vi "Resonator_response.vi"() -> ()   [LabVIEW 2020]
uses:
  <vilib>/Utility/file.llb/Write Delimited Spreadsheet (DBL).vi
  <instrlib>/Keysight PNA Series/Keysight PNA Series.lvlib
panel:
  out "State":T1(ring)=enum."Close"
  in  "PNA_control":T2={"Channel (1)"=1, "Start Frequency (Hz)"=6168700000.0, "Stop Frequency (Hz)"=6170700000.0, "Sweep Points (201)"=201, "Sweep Type (0: Linear)"=0, "Sweep Generation (1: Analog)"=1, "Bandwidth (Hz)"=100.0, "Average Count (1)"=200, "Enable Average "=TRUE, "Power"={"Attenuation (0 dB)"=0.0, "Power Level (0 dBm)"=-50.0, "Enable Auto Attenuation"=TRUE, "Enable RF Power"=TRUE, "Enable Power Slope"=FALSE, "Port (1)"=1, "Power Slope (0 dB/GHz)"=0.0}, "Enable Reduce IF Bandwidth "=TRUE, "Electrical delay"={"Unit (0: Meter)"=0, "Waveguide Cutoff Frequency (Hz)"=45000000.0, "Distance (0)"=0.0, "Medium "=0, "Delay (0 s)"=0.0}, "Measurement name"=["CH1_S12", "CH1_S22"], "Measurement Parameters (S11)"=["S12", "S22"]} {"Electrical delay"."Medium" items=["Coaxial", "Waveguide"]; "Electrical delay"."Unit (0: Meter)" items=["Meter", "Feet", "Inch"]; "Sweep Generation (1: Analog)" items=["Stepped", "Analog"]; "Sweep Type (0: Linear)" items=["Linear", "Logarithmic", "Power", "CW", "Segment", "Phase"]; "Stop Frequency (Hz)" format="%#_8g"; "Start Frequency (Hz)" format="%#_8g"}
  in  "Visa_Cluster":T3={"VNA visa"="GPIB0::16::INSTR", "MG369x visa"="GPIB0::8::INSTR", "Yokogawa visa"="GPIB0::1::INSTR"}
  in  "Save file path":path=path "D:/Sheng-Xiang_Lin/JPA_cooldown14/Fourth_resonator_dispersive_shift"
  in  "File_name":string="qubit"
  in  "Save?":bool=TRUE
  in  "Display format 1-2":T4={"Display Format 2"=3, "Display Format 1"=1} {"Display Format 1" items=["Magnitude Linear", "Magnitude Logarithmic", "Phase", "Unwrapped phase", "Imaginary", "Real", "Polar", "Smith Chart", "Smith Admittance", "SWR", "Group Delay", "Kelvin", "Fahrenheit", "Celsius"]; "Display Format 2" items=["Magnitude Linear", "Magnitude Logarithmic", "Phase", "Unwrapped phase", "Imaginary", "Real", "Polar", "Smith Chart", "Smith Admittance", "SWR", "Group Delay", "Kelvin", "Fahrenheit", "Celsius"]}
  in  "VNA_force_stop":bool
  out "average_times":i32=19
  in  "wait?":bool
  out "Magnitude":dbl[](array[numeric])=[-23.6737670898, -23.7385673523, -23.8055305481, -23.8746070862, -23.9425754547, -24.0142669678, -24.086517334, -24.1621208191, -24.2412757874, -24.3240642548, -24.410150528, -24.4976882935, -24.5875720978, -24.6802349091, -24.7777881622, -24.8763828278, -24.979177475, -25.0872688293, -25.2037525177, -25.3233108521, -25.4416027069, -25.5639820099, -25.704668045, -25.8504219055, -25.9997329712, -26.1532783508, -26.310962677, -26.474363327, -26.6452636719, -26.8241043091, -27.0116844177, -27.2097969055, -27.4203968048, -27.6485824585, -27.8864917755, -28.1318359375, -28.3951377869, -28.6704406738, -28.9638710022, -29.2743930817, -29.603849411, -29.9671974182, -30.3672046661, -30.7709980011, -31.1941585541, -31.6535701752, -32.1623039246, -32.7356109619, -33.3391723633, -34.0166893005, -34.7504501343, -35.5710372925, -36.4783821106, -37.4738388062, -38.6434822083, -40.0588035583, -41.7861747742, -43.9644699097, -46.8876876831, -51.4030303955, -60.4928474426, -57.0826530457, -49.7821121216, -45.7269706726, -42.9327430725, -40.7999610901, -39.0918464661, -37.6644554138, -36.410900116, -35.3036689758, -34.3229827881, -33.4435920715, -32.6499824524, -31.9220294952, -31.2542266846, -30.6332588196, -30.0641708374, -29.5344314575, -29.0330276489, -28.5691413879, -28.1316604614, -27.7197036743, -27.3364849091, -26.9709949493, -26.6234302521, -26.288225174, -25.977640152, -25.6853923798, -25.4085998535, -25.1478462219, -24.8998317719, -24.6655807495, -24.4424247742, -24.2275295258, -24.0214290619, -23.8225841522, -23.63697052, -23.4580116272, -23.3001346588, -23.1510028839, -23.0076026917, -22.8655033112, -22.7290058136, -22.5987110138, -22.4831619263, -22.3689022064, -22.2600975037, -22.1564464569, -22.0540332794, -21.9569740295, -21.8669834137, -21.7826919556, -21.7002334595, -21.6209335327, -21.5461406708, -21.4741287231, -21.4073295593, -21.3435554504, -21.2839221954, -21.2248191833, -21.1635513306, -21.1088104248, -21.0579814911, -21.0078163147, -20.9615936279, -20.9172554016, -20.8747119904, -20.833404541, -20.7956390381, -20.759349823, -20.7250919342, -20.6904773712, -20.6576309204, -20.6262359619, -20.5970096588, -20.5672588348, -20.5403385162, -20.5139713287, -20.4889431, -20.4652805328, -20.440788269, -20.4182872772, -20.3972473145, -20.3769702911, -20.3574924469, -20.338842392, -20.3210716248, -20.3047962189, -20.2892684937, -20.2742462158, -20.2597618103, -20.2454681396, -20.232049942, -20.2189407349, -20.2070941925, -20.1947593689, -20.1833267212, -20.1720867157, -20.1617012024, -20.1521492004, -20.1428623199, -20.1335334778, -20.1245746613, -20.1160011292, -20.1077804565, -20.0995311737, -20.0921134949, -20.0842552185, -20.0772380829, -20.0709438324, -20.0642986298, -20.0582752228, -20.0526847839, -20.0474853516, -20.0421714783, -20.0368518829, -20.0318584442, -20.0270271301, -20.0223388672, -20.0181751251, -20.0138206482, -20.0099639893, -20.0064086914, -20.0029449463, -19.9997406006, -19.9968338013, -19.993806839, -19.9911708832, -19.9880523682, -19.9856872559, -19.9832305908, -19.9805030823, -19.9782714844, -19.9759674072, -19.9742794037, -19.9721908569, -19.970664978, -19.9689235687, -19.9670543671, -19.9657402039, -19.9643135071] format="%#_8g"
  in  "Leave_pend":bool
  in  "Current_Value":T5={"Ch1 Intensity Graph"=array201x26[5226 elements], "Freq_Array"=array[201 elements], "Ch2 Intensity Graph"=array201x26[5226 elements], "Ch1"={"Magnitude"=array[201 elements], "Phase"=array[201 elements]}, "Ch2"={"Magnitude"=array[201 elements], "Phase"=array[201 elements]}, "Signal_power (dBm)"=2.0}
  in  "Limit_Cluster":T6={"Current_or_voltage_limit"=3.0, "Micro_freq_limit (GHz)"=4.71, "Micro_power_limit (dBm)"=0.0}
  in  "Force_stop":bool
  in  "Increment cluster":T7={"Yoko_Increment"=0.01, "Micro_Increment (GHz)"=0.0002, "Micro_power_inc (dBm)"=2.0}
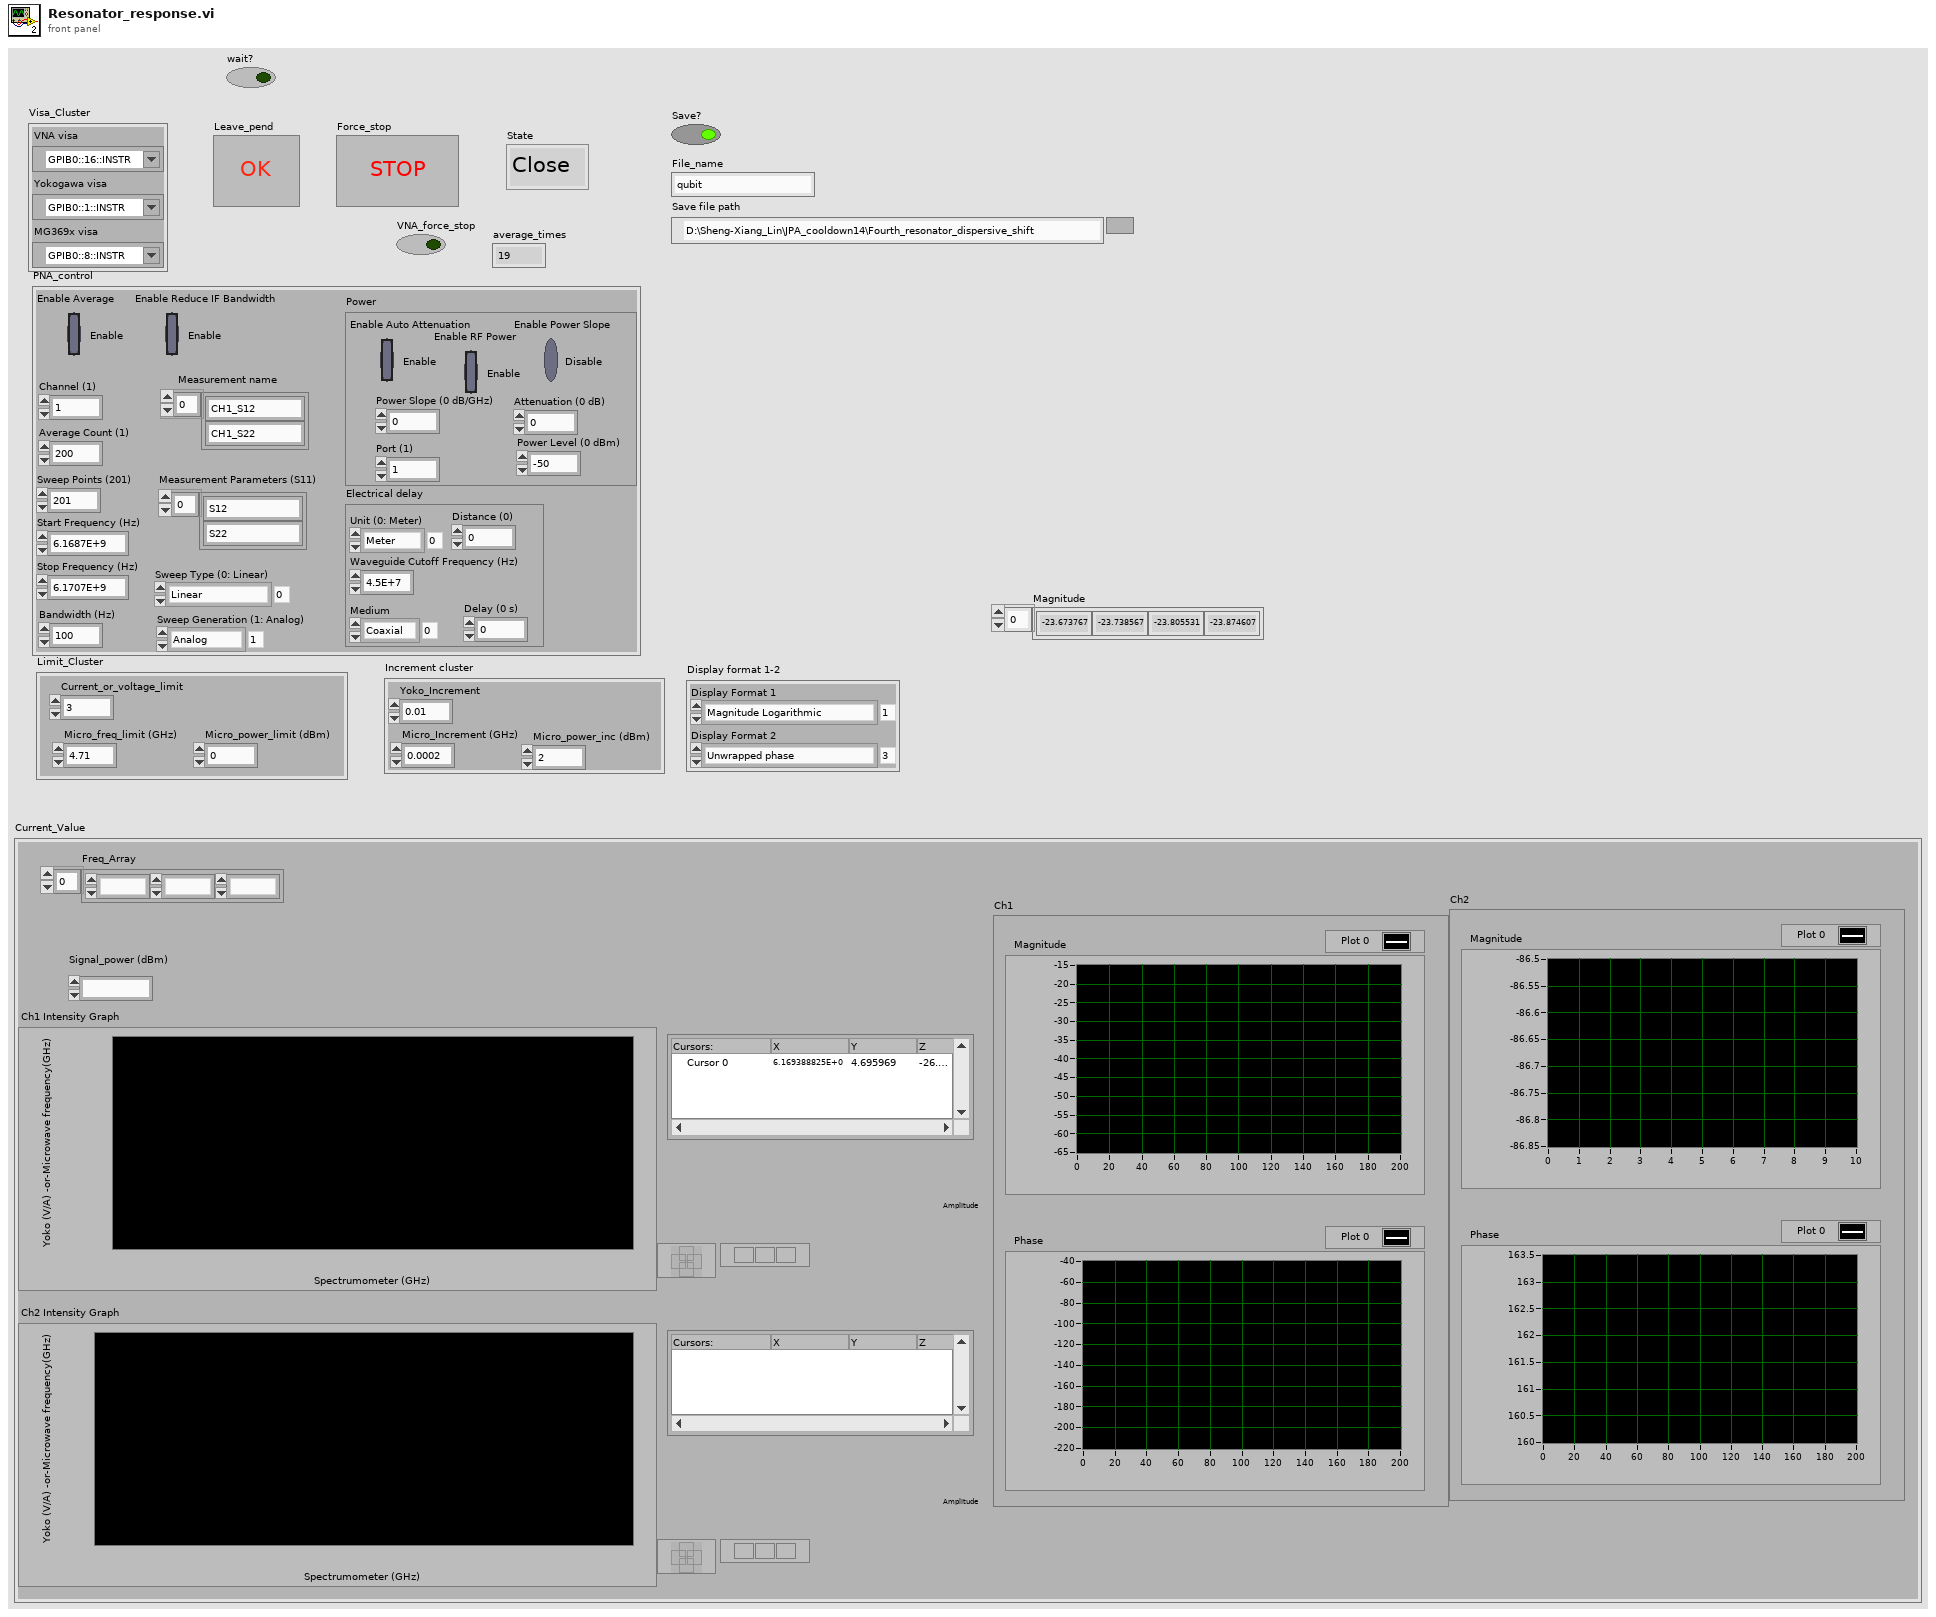
[diagram p1: front panel]
types:
  T1 = enum16{"Init", "Pend", "micro_scan", "Yogo_scan", "VNA_result", "Close", "Save_and_write", "VNA_configure"}
  T2 = cluster{"Channel (1)":i32, "Start Frequency (Hz)":dbl, "Stop Frequency (Hz)":dbl, "Sweep Points (201)":i32, "Sweep Type (0: Linear)":i32, "Sweep Generation (1: Analog)":i32, "Bandwidth (Hz)":dbl, "Average Count (1)":i32, "Enable Average ":bool, "Power":cluster{"Attenuation (0 dB)":dbl, "Power Level (0 dBm)":dbl, "Enable Auto Attenuation":bool, "Enable RF Power":bool, "Enable Power Slope":bool, "Port (1)":i32, "Power Slope (0 dB/GHz)":dbl}, "Enable Reduce IF Bandwidth ":bool, "Electrical delay":cluster{"Unit (0: Meter)":i32, "Waveguide Cutoff Frequency (Hz)":dbl, "Distance (0)":dbl, "Medium ":i32, "Delay (0 s)":dbl}, "Measurement name":string[], "Measurement Parameters (S11)":string[]}
  T3 = cluster{"VNA visa":refnum<visa-resource-name>, "MG369x visa":refnum<visa-resource-name>, "Yokogawa visa":refnum<visa-resource-name>}
  T4 = cluster{"Display Format 2":i32, "Display Format 1":i32}
  T5 = cluster{"Ch1 Intensity Graph":dbl[][], "Freq_Array":dbl[], "Ch2 Intensity Graph":dbl[][], "Ch1":cluster{"Magnitude":dbl[], "Phase":dbl[]}, "Ch2":cluster{"Magnitude":dbl[], "Phase":dbl[]}, "Signal_power (dBm)":dbl}
  T6 = cluster{"Current_or_voltage_limit":dbl, "Micro_freq_limit (GHz)":dbl, "Micro_power_limit (dBm)":dbl}
  T7 = cluster{"Yoko_Increment":dbl, "Micro_Increment (GHz)":dbl, "Micro_power_inc (dBm)":dbl}
  T8 = enum16{"Init", "Pend", "micro_scan", "Yogo_scan", "VNA_result", "Close"}
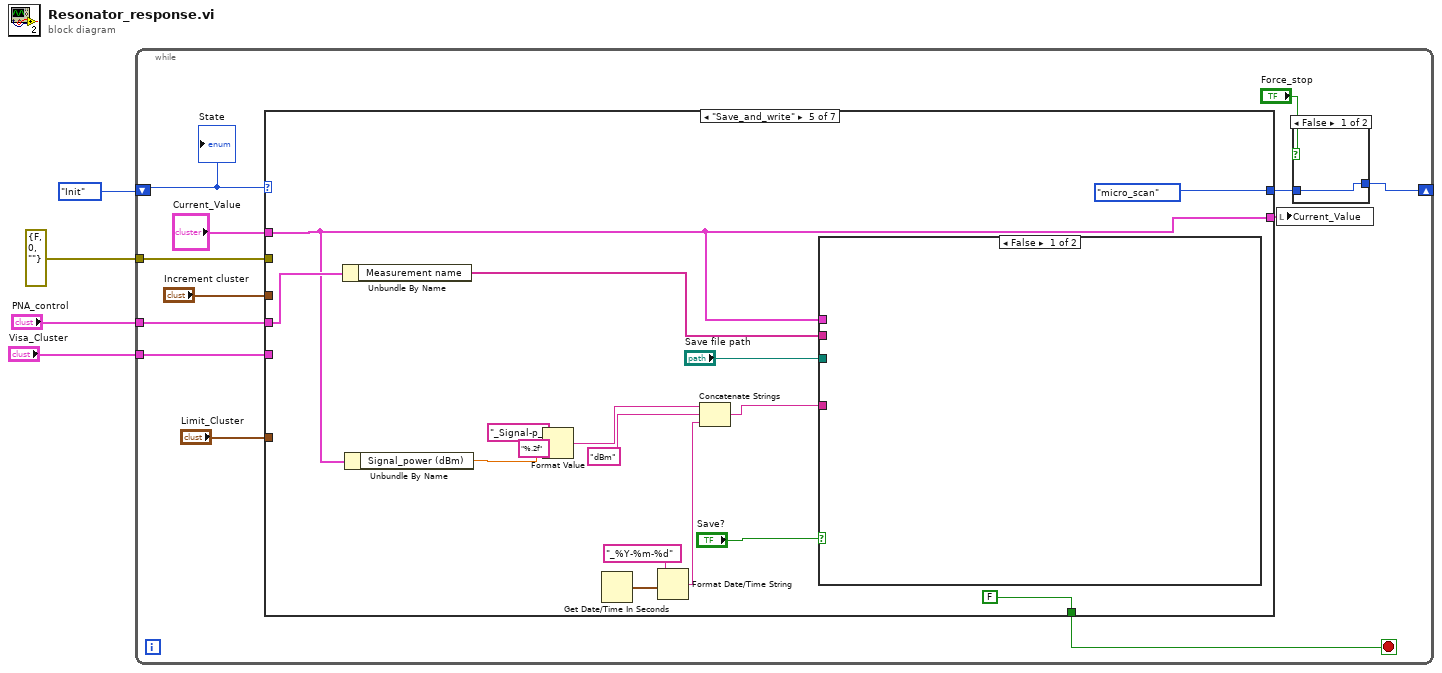
[diagram p0: block diagram]
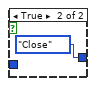
[diagram p2: hidden frame]
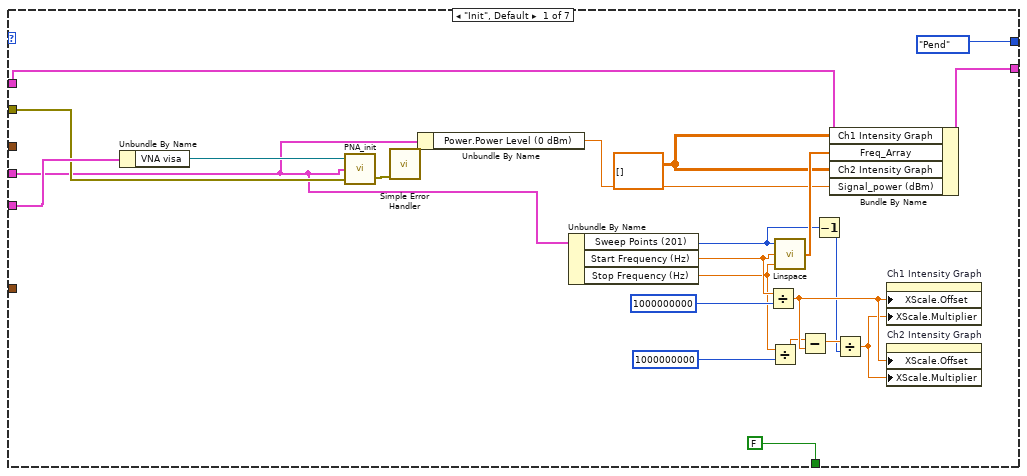
[diagram p3: hidden frame]
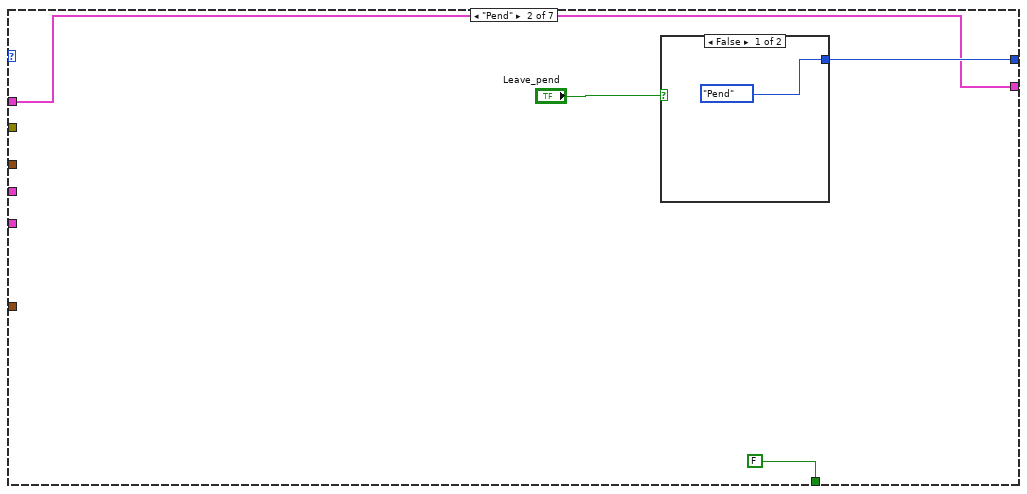
[diagram p4: hidden frame]
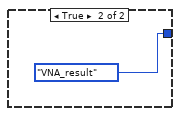
[diagram p5: hidden frame]
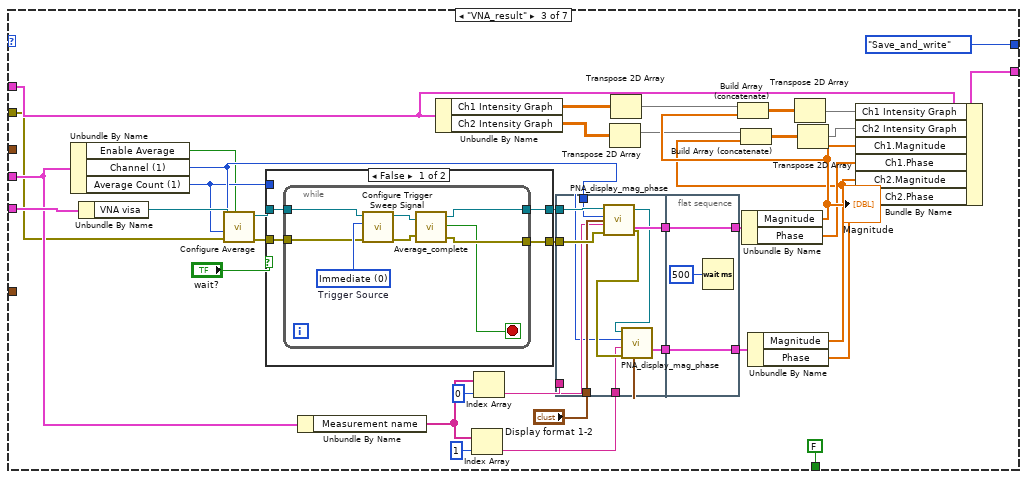
[diagram p6: hidden frame]
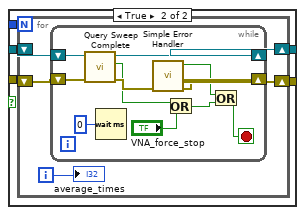
[diagram p7: hidden frame]
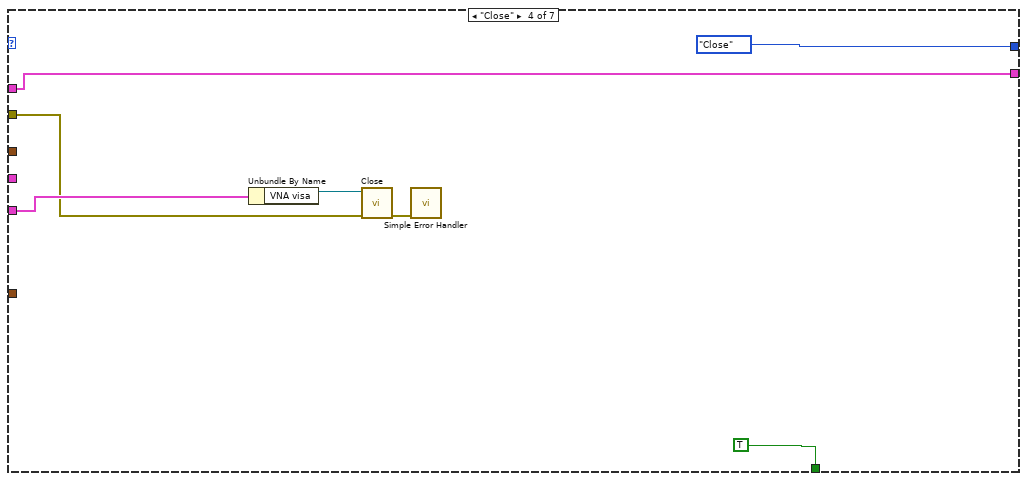
[diagram p8: hidden frame]
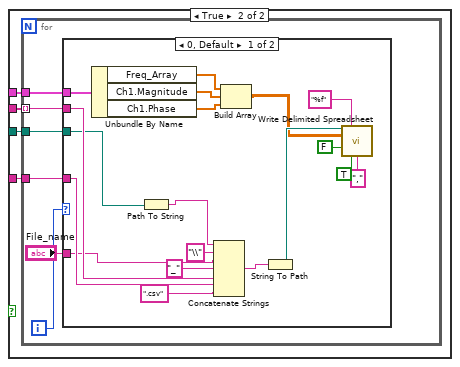
[diagram p9: hidden frame]
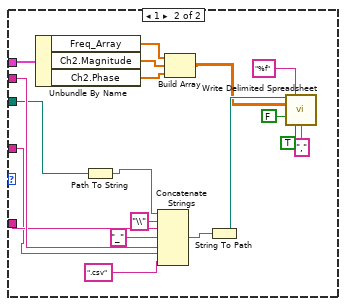
[diagram p10: hidden frame]
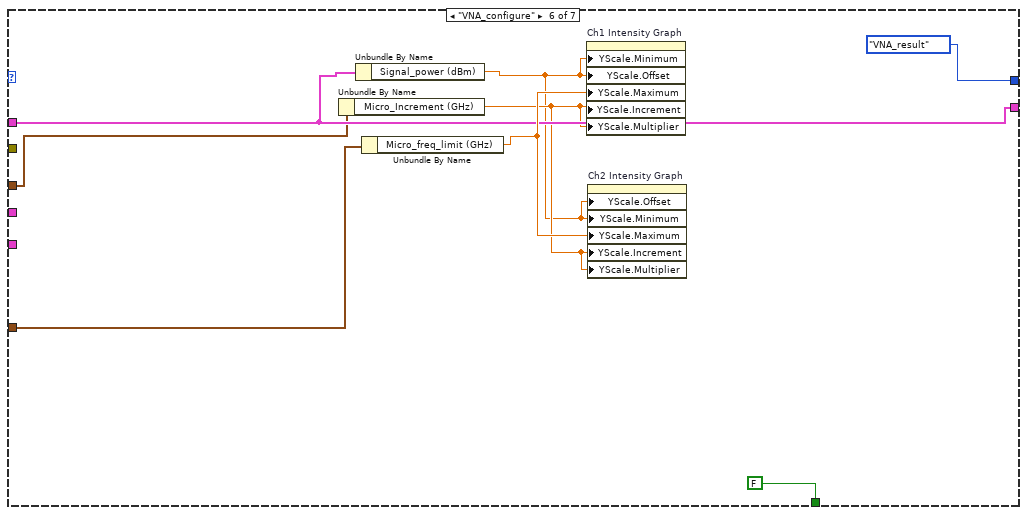
[diagram p11: hidden frame]
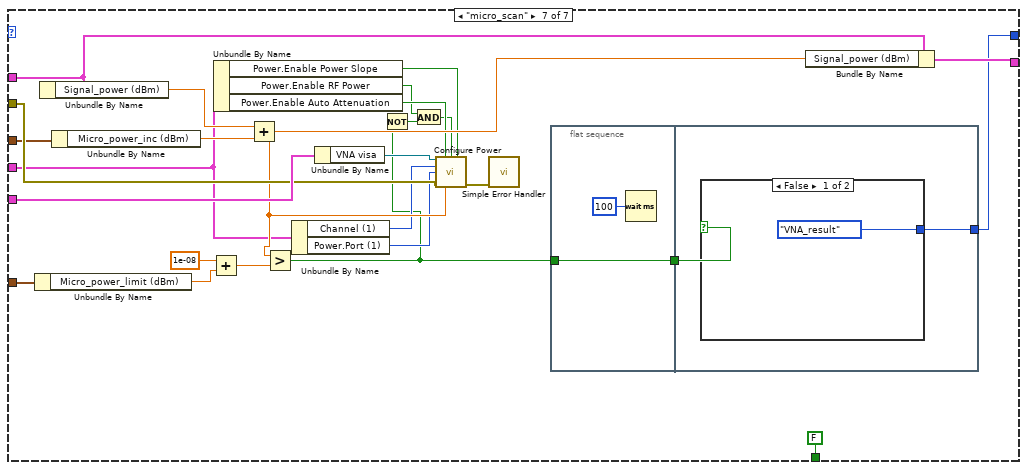
[diagram p12: hidden frame]
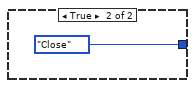
[diagram p13: hidden frame]
diagram:
  n1 = while {
    tunnel: errorcluster {"status"=FALSE, "code"=0, "source"=""} ("error in (no error)") -> [w16]
    tunnel: "Visa_Cluster" -> [w15]
    shift-right: [w10] -> _
    shift-left: T1."Init" ("State 2") -> [w5]
    tunnel: "PNA_control" -> [w7]
    stop <- w8 stop-if-true
    n2 = case shown="\"Save_and_write\"" w5 {
      tunnel: w16 -> [w38 _ w55 w134 _ _ w233]
      tunnel: w15 -> [w40 _ w84 w135 _ _ w234]
      tunnel: [T1."Pend" ("State 2") w44 T1."Save_and_write" ("State 2") T8."Close" ("State") T1."micro_scan" ("State 2") T1."VNA_result" ("State 2") w223] -> w9
      tunnel: [w36 w41 w75 w133 w140 w207 w225] -> w14
      tunnel: "Current_Value" -> [w37 w41 w82 w133 w140 w207 w220]
      tunnel: "Limit_Cluster" -> [_ _ _ _ _ w206 w227]
      tunnel: [FALSE FALSE FALSE TRUE FALSE FALSE FALSE] -> w8
      tunnel: w7 -> [w20 _ w58 _ w146 _ w217]
      tunnel: "Increment cluster" -> [_ _ _ _ _ w205 w232]
      frame "Init", Default {
        w32 = dbl[][] [] ("Intensity Graph")
        n3 = Unbundle By Name(w40) -> ("VNA visa"=w39:refnum<visa-resource-name>)
        n4 = call "PNA_init.vi"("error in (no error)"=w38, "PNA_control"=w20, "PNA_visa"=w39) -> ("error out"=w34:errorcluster)  [unwired: 1 out]
        n5 = call <vilib>:"Simple Error Handler.vi"("error in (no error)"=w34) -> ()  [unwired: 4 in, 5 out]
        n6 = Unbundle By Name(w20) -> ("Power.Power Level (0 dBm)"=w19:dbl)
        n7 = Unbundle By Name(w20) -> ("Sweep Points (201)"=w22:i32, "Start Frequency (Hz)"=w31:dbl, "Stop Frequency (Hz)"=w28:dbl)
        n8 = Divide(x=w31, y=i64 1000000000) -> (x/y=w27:dbl)
        n9 = Divide(x=w28, y=i64 1000000000) -> (x/y=w26:dbl)
        n10 = call "Linspace.vi"("Stop_value"=w28, "Start_value"=w31, "Num"=w22) -> ("Output_array"=w33:dbl[])
        n11 = Subtract(x=w26, y=w27) -> (x-y=w25:dbl)
        n12 = Decrement(x=w22) -> (x-1=w23:i32)
        n13 = Bundle By Name(cluster=w37, "Ch1 Intensity Graph"=w32, "Freq_Array"=w33, "Ch2 Intensity Graph"=w32, "Signal_power (dBm)"=w19) -> (w36:T5)
        n14 = Divide(x=w25, y=w23) -> (x/y=w24:dbl)
        n15 = property on="Ch1 Intensity Graph" class="IntGraph (strict)"("XScale.Offset"=w27, "XScale.Multiplier"=w24) -> ()  [unwired: 2 in, 2 out]
        n16 = property on="Ch2 Intensity Graph" class="IntGraph (strict)"("XScale.Offset"=w27, "XScale.Multiplier"=w24) -> ()  [unwired: 2 in, 2 out]
      }
      frame "Pend" {
        n17 = case shown="False" "Leave_pend" {
          tunnel: [T1."Pend" ("State 2") T1."VNA_result" ("State 2")] -> w44
          frame False {
          }
          frame True {
          }
        }
      }
      frame "VNA_result" {
        n18 = Unbundle By Name(w58) -> ("Enable Average"=w51:bool, "Channel (1)"=w53:i32, "Average Count (1)"=w52:i32)
        n19 = Unbundle By Name(w84) -> ("VNA visa"=w54:refnum<visa-resource-name>)
        n20 = call <instrlib>:"Configure Average.vi"("Enable Average (F: Disable)"=w51, "error in (no error)"=w55, "Average Count (1)"=w52, "Channel (1)"=w53, "VISA resource name"=w54) -> ("error out"=w56:errorcluster, "VISA resource name out"=w57:refnum<visa-resource-name>)  [unwired: 5 in]
        n21 = case shown="False" "wait?" {
          tunnel: [w101 w114] -> w78
          tunnel: [w100 w113] -> w77
          tunnel: w57 -> [w99 w112]
          tunnel: w56 -> [w98 w111]
          tunnel: w52 -> [_ w110]
          frame False {
            n22 = while {
              tunnel: [w108] -> w101
              tunnel: [w107] -> w100
              tunnel: w99 -> [w103]
              tunnel: w98 -> [w102]
              stop <- w106 stop-if-true
              w109 = 0 items=["Immediate", "External", "Manual"]  # Trigger Source
              n23 = call <instrlib>:"Configure Trigger Sweep Signal.vi"("error in (no error)"=w102, "Trigger Source (0: Immediate)"=w109, "VISA resource name"=w103) -> ("error out"=w105:errorcluster, "VISA resource name out"=w104:refnum<visa-resource-name>)  [unwired: 7 in]
              n24 = call "Average_complete.vi"("VISA resource name"=w104, "error in (no error)"=w105) -> ("VISA resource name out"=w108:refnum<visa-resource-name>, "Average Complete"=w106:bool, "error out"=w107:errorcluster)
            }
          }
          frame True {
            n25 = for {
              N: w110 -> [_]
              shift-right: [w119] -> w114
              shift-left: w112 -> [w116]
              shift-right: [w118] -> w113
              shift-left: w111 -> [w115]
              i -> [w117]
              n26 = while {
                shift-right: [w125] -> w118
                shift-left: w115 -> [w130]
                shift-right: [w128] -> w119
                shift-left: w116 -> [w129]
                stop <- w123 stop-if-true
                n27 = call <instrlib>:"Query Sweep Complete.vi"("error in (no error)"=w130, "VISA resource name"=w129) -> ("error out"=w126:errorcluster, "Sweep Complete"=w121:bool, "VISA resource name out"=w128:refnum<visa-resource-name>)  [unwired: 7 in]
                n28 = Wait (ms)(milliseconds to wait=u32 0) -> ()  [unwired: 1 out]
                n29 = call <vilib>:"Simple Error Handler.vi"("error in (no error)"=w126) -> ("error?"=w124:bool, "error out"=w125:errorcluster)  [unwired: 4 in, 3 out]
                n30 = Or(x=w121, y="VNA_force_stop") -> (x .or. y?=w122:bool)
                n31 = Or(x=w124, y=w122) -> (x .or. y?=w123:bool)
              }
              "average_times" <- w117
            }
          }
        }
        n32 = Unbundle By Name(w58) -> ("Measurement name"=w63:string[])
        n33 = Unbundle By Name(w82) -> ("Ch1 Intensity Graph"=w81:dbl[][], "Ch2 Intensity Graph"=w69:dbl[][])
        n34 = Index Array(array=w63, index=1) -> (element=w59:string)
        n35 = Index Array(array=w63, index=0) -> (element=w60:string)
        n36 = flat-sequence {
          tunnel: w78 -> [w94]
          tunnel: w77 -> [w93]
          tunnel: "Display format 1-2" -> [w89]
          tunnel: w60 -> [w87]
          tunnel: w59 -> [w86]
          tunnel: w53 -> [w85]
          tunnel: [w92] -> w49
          tunnel: [w88] -> w48
          tunnel: [w96] -> w71
          tunnel: [w97] -> w76
          tunnel: w49 -> [w97]
          tunnel: w48 -> [w96]
          frame #0 {
            n37 = call "PNA_display_mag_phase.vi"("VISA resource name"=w94, "Channel (1)"=w85, "Measurement Name (CH1_S11)"=w87, "error in (no error)"=w93, "Display format 1-2"=w89) -> ("VISA resource name out"=w91:refnum<visa-resource-name>, "Cluster"=w92:cluster{"Magnitude":dbl[], "Phase":dbl[]}, "error out"=w90:errorcluster)
            n38 = call "PNA_display_mag_phase.vi"("VISA resource name"=w91, "Channel (1)"=w85, "Measurement Name (CH1_S11)"=w86, "error in (no error)"=w90, "Display format 1-2"=w89) -> ("Cluster"=w88:cluster{"Magnitude":dbl[], "Phase":dbl[]})  [unwired: 2 out]
          }
          frame #1 {
            n39 = Wait (ms)(milliseconds to wait=u32 500) -> ()  [unwired: 1 out]
          }
        }
        n40 = Transpose 2D Array(2D array=w69) -> (transposed array=w66:dbl[][])
        n41 = Transpose 2D Array(2D array=w81) -> (transposed array=w80:dbl[][])
        n42 = Unbundle By Name(w76) -> ("Magnitude"=w74:dbl[], "Phase"=w73:dbl[])
        "Magnitude" <- w74
        n43 = Build Array (concatenate)(w80, w74) -> (w79:dbl[][])
        n44 = Unbundle By Name(w71) -> ("Magnitude"=w64:dbl[], "Phase"=w70:dbl[])
        n45 = Build Array (concatenate)(w66, w64) -> (w67:dbl[][])
        n46 = Transpose 2D Array(2D array=w79) -> (transposed array=w68:dbl[][])
        n47 = Transpose 2D Array(2D array=w67) -> (transposed array=w65:dbl[][])
        n48 = Bundle By Name(cluster=w82, "Ch1 Intensity Graph"=w68, "Ch2 Intensity Graph"=w65, "Ch1.Magnitude"=w74, "Ch1.Phase"=w73, "Ch2.Magnitude"=w64, "Ch2.Phase"=w70) -> (w75:T5)
      }
      frame "Close" {
        n49 = Unbundle By Name(w135) -> ("VNA visa"=w136:refnum<visa-resource-name>)
        n50 = call <instrlib>:"Close.vi"("error in (no error)"=w134, "VISA resource name"=w136) -> ("error out"=w137:errorcluster)  [unwired: 9 in]
        n51 = call <vilib>:"Simple Error Handler.vi"("error in (no error)"=w137) -> ()  [unwired: 4 in, 5 out]
      }
      frame "Save_and_write" {
        n52 = Unbundle By Name(w146) -> ("Measurement name"=w145:string[])
        n53 = Unbundle By Name(w140) -> ("Signal_power (dBm)"=w151:dbl)
        n54 = Format Value(string ("")="_Signal-p_", format string="%.2f", value (0)=w151) -> (output string=w150:string)
        n55 = Get Date/Time In Seconds() -> (seconds since 1Jan1904=w148:timestamp)
        n56 = Format Date/Time String(time format string (%c)="_%Y-%m-%d", seconds (now)=w148) -> (date/time string=w138:string)  [unwired: 1 in]
        n57 = Concatenate Strings(w150, "dBm" ("string"), w138) -> (w144:string)
        n58 = case shown="False" "Save?" {
          tunnel: w140 -> [_ w157]
          tunnel: w145 -> [_ w156]
          tunnel: w144 -> [_ w155]
          tunnel: "Save file path" -> [_ w154]
          frame False {
          }
          frame True {
            n59 = for {
              tunnel: w157 -> [w162]
              tunnel: w156 -> [w161] mode=indexing
              tunnel: w155 -> [w160]
              tunnel: w154 -> [w159]
              i -> [w163]
              n60 = case shown="0, Default" w163 {
                tunnel: w162 -> [w168 w187]
                tunnel: w161 -> [w167 w186]
                tunnel: w160 -> [w166 w183]
                tunnel: w159 -> [w165 w185]
                tunnel: "File_name" -> [w164 w184]
                frame 0, Default {
                  n61 = Unbundle By Name(w168) -> ("Freq_Array"=w174:dbl[], "Ch1.Magnitude"=w172:dbl[], "Ch1.Phase"=w173:dbl[])
                  n62 = Path To String(path=w165) -> (string=w169:string)
                  n63 = Concatenate Strings(w169, "\\" ("string"), w164, "_" ("input 2"), w167, w166, ".csv" ("input 3")) -> (w176:string)
                  n64 = Build Array(w174, w172, w173) -> (w171:dbl[][])
                  n65 = String To Path(string=w176) -> (path=w175:path)
                  n66 = call-poly <vilib>:"Write Delimited Spreadsheet.vi"("file path (dialog if empty)"=w175, "format (%.3f)"="%f", "2D data"=w171, "append to file? (new file:F)"=FALSE, "transpose? (no:F)"=TRUE, "delimiter (\\t)"="," ("delimiter (\\t)")) -> ()  [unwired: 8 in, 2 out]
                }
                frame 1 {
                  n67 = Unbundle By Name(w187) -> ("Freq_Array"=w193:dbl[], "Ch2.Magnitude"=w191:dbl[], "Ch2.Phase"=w192:dbl[])
                  n68 = Path To String(path=w185) -> (string=w188:string)
                  n69 = Concatenate Strings(w188, "\\" ("string"), w184, "_" ("input 2"), w186, w183, ".csv" ("input 3")) -> (w195:string)
                  n70 = Build Array(w193, w191, w192) -> (w190:dbl[][])
                  n71 = String To Path(string=w195) -> (path=w194:path)
                  n72 = call-poly <vilib>:"Write Delimited Spreadsheet.vi"("file path (dialog if empty)"=w194, "format (%.3f)"="%f", "2D data"=w190, "append to file? (new file:F)"=FALSE, "transpose? (no:F)"=TRUE, "delimiter (\\t)"="," ("delimiter (\\t)")) -> ()  [unwired: 8 in, 2 out]
                }
              }
            }
          }
        }
      }
      frame "VNA_configure" {
        n73 = Unbundle By Name(w205) -> ("Micro_Increment (GHz)"=w204:dbl)
        n74 = Unbundle By Name(w207) -> ("Signal_power (dBm)"=w203:dbl)
        n75 = Unbundle By Name(w206) -> ("Micro_freq_limit (GHz)"=w208:dbl)
        n76 = property on="Ch1 Intensity Graph" class="IntGraph (strict)"("YScale.Minimum"=w203, "YScale.Offset"=w203, "YScale.Maximum"=w208, "YScale.Increment"=w204, "YScale.Multiplier"=w204) -> ()  [unwired: 2 in, 2 out]
        n77 = property on="Ch2 Intensity Graph" class="IntGraph (strict)"("YScale.Offset"=w203, "YScale.Minimum"=w203, "YScale.Maximum"=w208, "YScale.Increment"=w204, "YScale.Multiplier"=w204) -> ()  [unwired: 2 in, 2 out]
      }
      frame "micro_scan" {
        n78 = Unbundle By Name(w227) -> ("Micro_power_limit (dBm)"=w226:dbl)
        n79 = Unbundle By Name(w220) -> ("Signal_power (dBm)"=w230:dbl)
        n80 = Unbundle By Name(w232) -> ("Micro_power_inc (dBm)"=w231:dbl)
        n81 = Add(x=1e-08, y=w226) -> (x+y=w229:dbl)
        n82 = Unbundle By Name(w217) -> ("Power.Enable Power Slope"=w218:bool, "Power.Enable RF Power"=w213:bool, "Power.Enable Auto Attenuation"=w219:bool)
        n83 = Add(x=w230, y=w231) -> (x+y=w224:dbl)
        n84 = Greater?(x=w224, y=w229) -> (0:w211:bool)
        n85 = Unbundle By Name(w217) -> ("Channel (1)"=w216:i32, "Power.Port (1)"=w215:i32)
        n86 = Unbundle By Name(w234) -> ("VNA visa"=w235:refnum<visa-resource-name>)
        n87 = Not(x=w211) -> (.not. x?=w212:bool)
        n88 = And(x=w213, y=w212) -> (x .and. y?=w210:bool)
        n89 = call <instrlib>:"Configure Power.vi"("VISA resource name"=w235, "Enable Auto Attenuation (T: Enable)"=w219, "Enable RF Power (T: Enable)"=w210, "Enable Power Slope (F: Disable)"=w218, "Channel (1)"=w216, "Port (1)"=w215, "error in (no error)"=w233, "Power Level (0 dBm)"=w224) -> ("error out"=w214:errorcluster)  [unwired: 6 in, 1 out]
        n90 = call <vilib>:"Simple Error Handler.vi"("error in (no error)"=w214) -> ()  [unwired: 4 in, 5 out]
        n91 = flat-sequence {
          tunnel: w211 -> [w237]
          tunnel: [w237] -> w221
          tunnel: [w238] -> w223
          tunnel: w221 -> [w239]
          frame #0 {
            n92 = Wait (ms)(milliseconds to wait=u32 100) -> ()  [unwired: 1 out]
          }
          frame #1 {
            n93 = case shown="False" w239 {
              tunnel: [T1."VNA_result" ("State 2") T1."Close" ("State 2")] -> w238
              frame False {
              }
              frame True {
              }
            }
          }
        }
        n94 = Bundle By Name(cluster=w220, "Signal_power (dBm)"=w224) -> (w225:T5)
      }
    }
    n95 = local write "Current_Value"(w14) -> ()
    n96 = case shown="False" "Force_stop" {
      tunnel: [w17 T8."Close" ("State")] -> w10
      tunnel: w9 -> [w17 _]
      frame False {
      }
      frame True {
      }
    }
    "State" <- w5
  }
